vi "JSON Global.vi"(7 "Write (F)":bool, 11 "JSON In":T1) -> (3 "JSON Out":T1)   [LabVIEW 2019]
uses:
  Type Defs/JSON_Tank.ctl
  Type Defs/JSON_Channel.ctl
  Type Defs/JSON_Pump.ctl
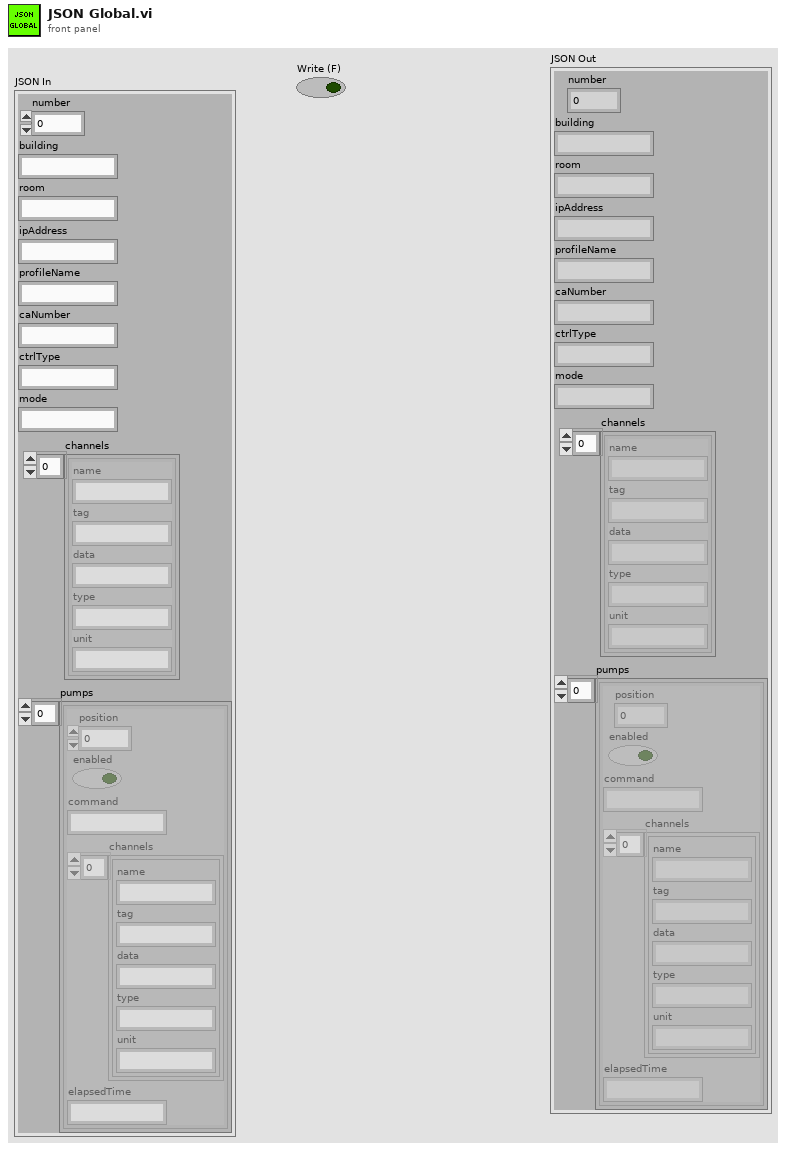
[diagram p1: front panel]
types:
  T1 = typedef "JSON_Tank.ctl" = cluster{"number":u16, "building":string, "room":string, "ipAddress":string, "profileName":string, "caNumber":string, "ctrlType":string, "mode":string, "channels":T2[], "pumps":T3[]}
  T2 = typedef "JSON_Channel.ctl" = cluster{"name":string, "tag":string, "data":string, "type":string, "unit":string}
  T3 = typedef "JSON_Pump.ctl" = cluster{"position":u8, "enabled":bool, "command":string, "channels":T2[], "elapsedTime":string}
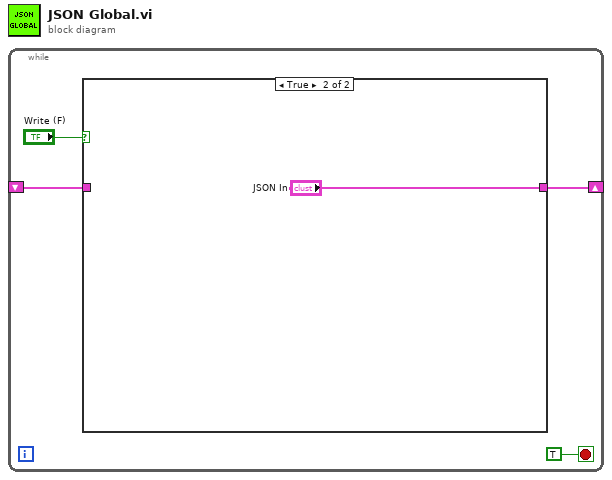
[diagram p0: block diagram]
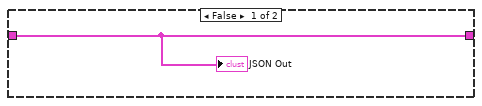
[diagram p2: hidden frame]
diagram:
  n1 = while {
    shift-right: [w2] -> _
    shift-left: _ -> [w1]
    stop <- TRUE stop-if-true
    n2 = case shown="True" "Write (F)" {
      tunnel: [w5 "JSON In"] -> w2
      tunnel: w1 -> [w5 _]
      frame False {
        "JSON Out" <- w5
      }
      frame True {
      }
    }
  }
